vi "全局 1.vi"() -> ()   [LabVIEW 2018]
panel:
  in  "选项卡控件":enum32{"系统", "PLC", "VISON", "Mdbus", "中英文"}(tab)
  out "Exit 2":bool
  out "Exit 1":bool
  out "产品名称0":string
  out "物料编号4":string
  out "物料编号3":string
  out "产品名称2":string
  in  "系统时间":timestamp
  out "物料编号2":string
  out "机台编号":string
  out "物料编号1":string
  out "产线编号":string
  out "Login PW":dbl[](array[numeric])=[12.34, -43.21] format="%.2f"
  out "Login":i32
  out "CCIEFB Slave IP":string="192.168.3.2"
  out "ROBOT PORT":u16 format="%08x"
  out "ROBOT IP":string
  out "PLC PORT":u16 format="%08x"
  out "PLC IP":string
  out "ini文件":path
  out "产品名称1":string
  out "Exit":bool
  out "当前档位":u16
  out "PCTOUTAC远程/本地控制":bool
  out "PCTOUTAC读取目标挡位数据完成":bool
  out "配方编号":u16
  out "动作数量":string
  out "备注":string
  out "样品编号":string
  out "零件编号":string
  out "零件名称":string
  out "项目编号":string
  out "时间":sgl
  out "1# 时间数组簇":cluster{"Time":i32[]}
  out "1# 方向数组簇":T1
  out "PCTOUTAC换挡不成功":bool
  out "PCTOUTAC换挡到位":bool
  out "PCTOUTAC正在换挡":bool
  out "PCTOUTAC急停":bool
  out "PCTOUTAC学习":bool
  out "PCTOUTAC故障":bool
  out "PCTOUTAC运行/停机":bool
  out "PCTOPLC读配方结束":bool
  out "PCTOPLC下发配方参数完成":bool
  out "PCTOPLC发送启动信号":bool
  out "PCTOPLC收到NO/OFF":bool
  out "PCTOPLC读取配方完成":bool
  out "PCTOPLC下发任务完成":bool
  out "PCTOPLC保存完成":bool
  out "PCTOPLC就绪":bool
  out "PLC状态位":T2
  out "PLC档位序号":T3
  out "PLC采集值":T4
  out "检测序号":u16
  out "PLC结果":T5
  out "PLC状态":T6
  out "力":sgl[](array[numeric]) format="%.4f"
  out "检测步骤":T7
  out "PLC检测值":T8 {"3#LED电压" format="%.2f"; "3#LED电流" format="%.2f"; "3#风门开电压" format="%.2f"; "3#风门闭电压" format="%.2f"; "3#稳定压力" format="%.1f"; "3#当前压力" format="%.1f"; "3#稳定泄漏量" format="%.2f"; "3#当前泄漏量" format="%.2f"; "2#LED电压" format="%.2f"; "2#LED电流" format="%.2f"; "2#风门开电压" format="%.2f"; "2#风门闭电压" format="%.2f"; "2#稳定压力" format="%.1f"; "2#当前压力" format="%.1f"; "2#稳定泄漏量" format="%.2f"; "2#当前泄漏量" format="%.2f"; "1#LED电压" format="%.2f"; "1#LED电流" format="%.2f"; "1#风门开电压" format="%.2f"; "1#风门闭电压" format="%.2f"; "1#稳定压力" format="%.1f"; "1#当前压力" format="%.1f"; "1#稳定泄漏量" format="%.2f"; "1#当前泄漏量" format="%.2f"}
  out "高低配":i16
  out "PLC检测参数":T9 {"INV快速变化量" format="%.2f"; "INV慢速变化量" format="%.2f"; "INV变化周期" format="%.1f"; "INV初始频率" format="%.2f"; "伺服速度" format="%.1f"; "气压稳定时间" format="%.1f"; "LED电流下限" format="%.2f"; "LED电流上限" format="%.2f"; "风门开电压下限" format="%.2f"; "风门开电压上限" format="%.2f"; "风门闭电压下限" format="%.2f"; "风门闭电压上限" format="%.2f"; "压力下限" format="%.1f"; "压力上限" format="%.1f"; "泄漏量上限" format="%.2f"; "轮盘预压力" format="%.1f"}
  out "PC状态":cluster{"PLC就绪":bool, "空动作中":bool}
  out "总测试次数":i16
  out "3#视觉检测":u16[](array[numeric])
  out "2#视觉检测":u16[](array[numeric])
  out "1#视觉检测":u16[](array[numeric])
  out "PCTOUTAC参数":i16[](array[numeric])
  out "UTACTOPLC复位到原点":bool
  out "UTACTOPLC急停":bool
  out "UTACTOPLC故障复位":bool
  out "UTACTOPLC故障":bool
  out "UTACTOPLC运行/停机":bool
  out "终止序号":i16
  out "起始序号":i16
  out "UTAC设定参数":i16[](array[numeric])
  out "C-N编辑设定参数":string[](array[string])=["Delay_Time", "Acceleration_time", "Deceleration time", "X_Upper_value", "X_Lowerr_value", "Y_Upper_value", "Y_Lowerr_value", "X_displacement", "Y_displacement", "Repeat_number", "Definite_write", "Exit"]
  out "C-N编辑配方":string[](array[string])=["Recipe_number", "Detailed_location", "Explain", "Definite_write", "Exit"]
  out "C-N远程/本地":string[](array[string])=["Remote/Local", "Remote/Local Control"]
  out "C-N当前档位":string[](array[string])=["PCTOUTAC_Current_Shifter", "Current_Shifter"]
  out "C-N目标档位":string[](array[string])=["UTACTOPC_Target_Shifter", "Target_Shifter"]
  out "C-N设置":string[](array[string])=["Set", "Exit", "Edit_Recipe", "Edit_SetParameter"]
  out "C-NDI信号":string[](array[string])=["PCTOUTAC_DI_Signal", "Run/Stop", "Breakdown", "study", "Stop", "Is_Shifter", "Shifter_Succeed", "Shifter_FaildShifter"]
  out "C-NDO信号":string[](array[string])=["UTACTOPC_DO_Signal", "Run/Stop", "Breakdown", "Breakdown_Reset", "Stop", "Reset_To_origin"]
  out "C-N项目信息":string[](array[string])=["ltem_Information", "ltem_no", "Part_Name", "Part_No", "Sample_No", "Remark", "Action_Number", "Total_Test_Number", "Set"]
  # "PCTOUTAC"
  # "PCTOPLC"
  # "UTACTOPLC"
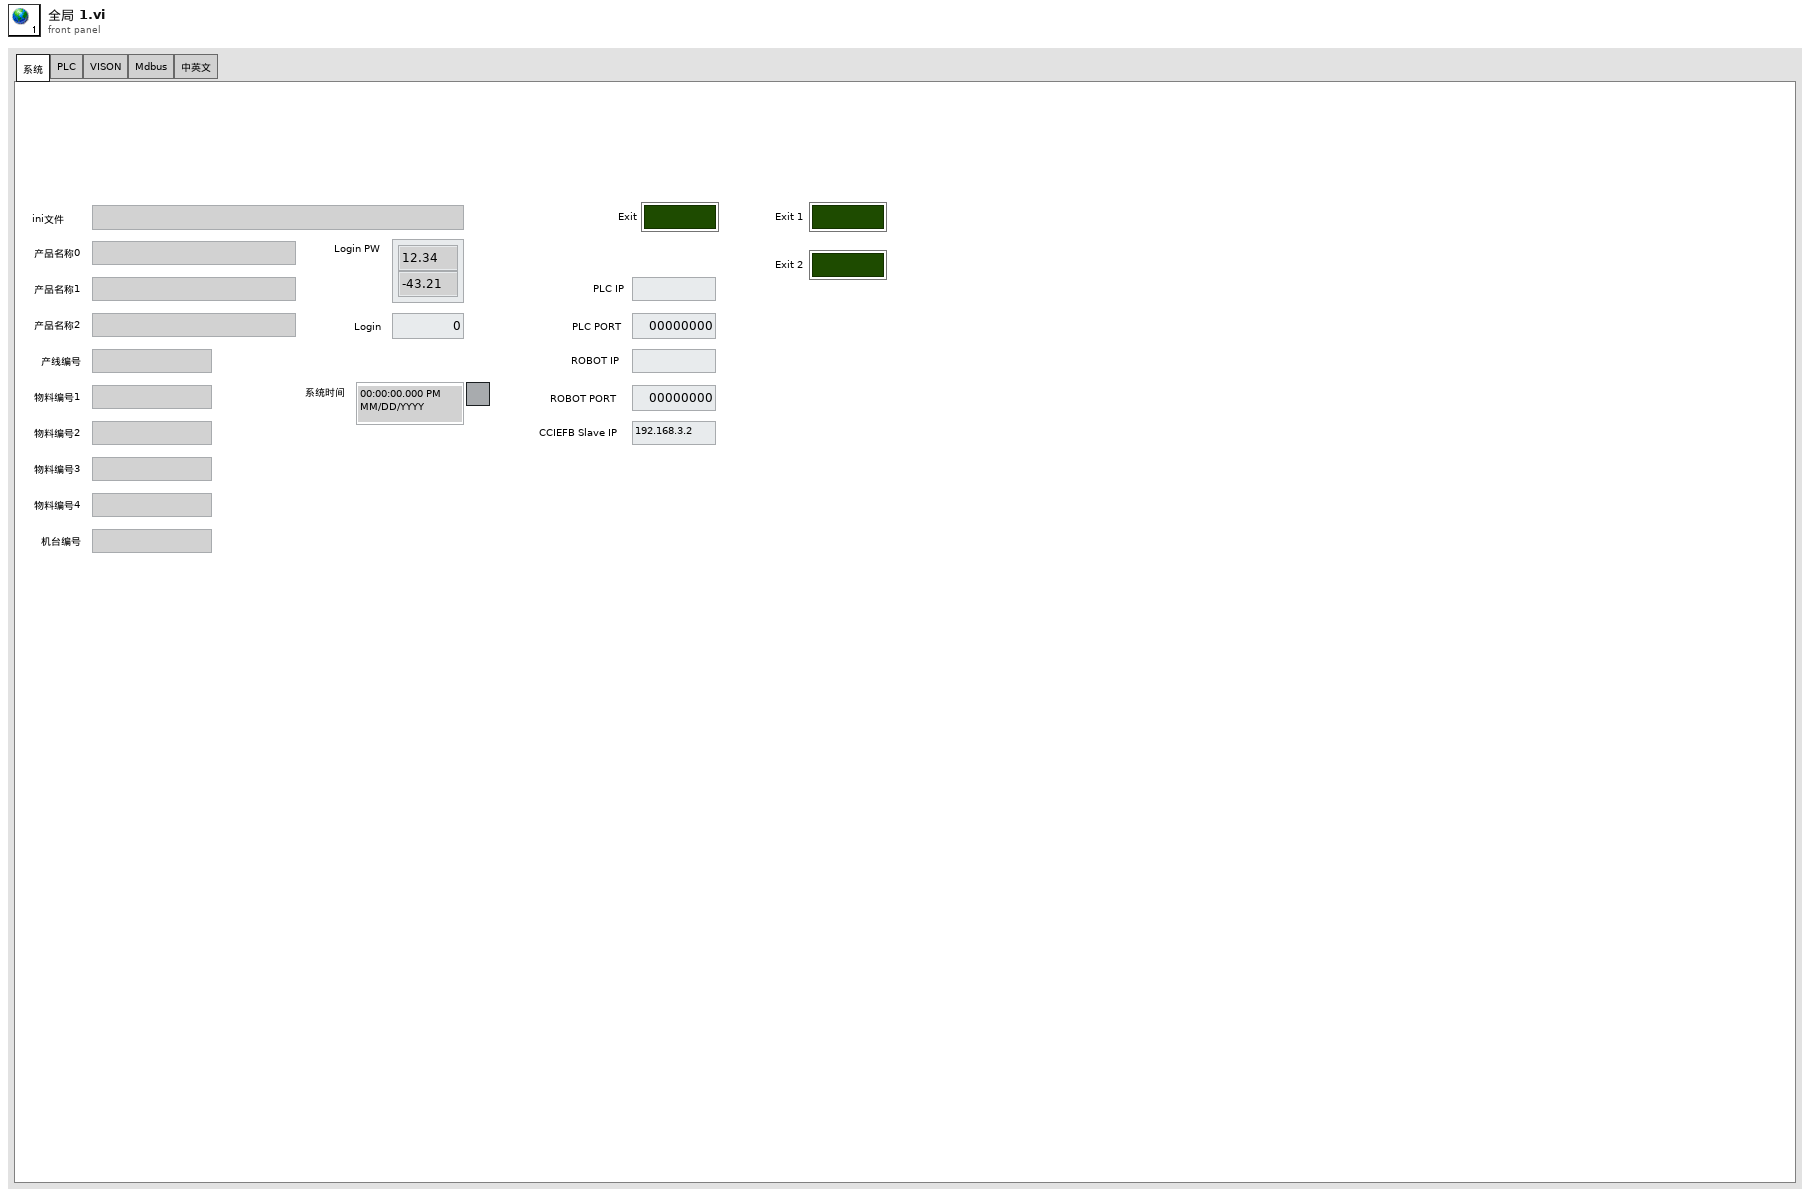
[diagram p1: front panel]
types:
  T1 = cluster{"Fx":sgl[], "Fy":sgl[], "Dx":sgl[], "Dy":sgl[]}
  T2 = cluster{"就绪":bool, "运行/停机":bool, "故障":bool, "学习":bool, "急停":bool, "正在换挡":bool, "换挡到位":bool, "换挡不成功":bool, "备用1":bool, "保存开始":bool, "等待下发任务":bool, "允许读取配方":bool, "开始采集数据":bool, "时间ON/OFF":bool, " 收到启动信号":bool, "结束采集信号":bool, "读配方参数ON/OFF":bool, "允许下发配方参数":bool}
  T3 = cluster{"挡位N1所在序号":sgl, "挡位1所在序号":sgl, "挡位N1所在序号":sgl, "挡位2所在序号":sgl, "挡位N1所在序号":sgl, " 挡位N2所在序号":sgl, "挡位3所在序号":sgl, "挡位N2所在序号":sgl, "挡位4所在序号":sgl, " 挡位N2所在序号":sgl, "挡位N3所在序号":sgl, "挡位5所在序号":sgl, "挡位N3所在序号":sgl, "挡位6所在序号":sgl, "挡位N3所在序号":sgl, "挡位N4所在序号":sgl, " 挡位7所在序号":sgl, " 挡位N4所在序号":sgl, "挡位8所在序号":sgl, "挡位N4所在序号":sgl, " 挡位N5所在序号":sgl, "挡位9所在序号":sgl, "挡位N5所在序号":sgl, " 挡位10所在序号":sgl}
  T4 = cluster{"X方向力值":sgl, "Y方向力值":sgl, "X方向位移值":sgl, "Y方向位移值":sgl}
  T5 = cluster{"1#泄漏量":bool, "1#风门闭电压":bool, "1#风门开电压":bool, "1#LED电压":bool, "1#LED电流":bool, "外观结果":bool, "2#泄漏量":bool, "2#风门闭电压":bool, "2#风门开电压":bool, "2#LED电压":bool, "2#LED电流":bool, "3#泄漏量":bool, "3#风门闭电压":bool, "3#风门开电压":bool, "3#LED电压":bool, "3#LED电流":bool}
  T6 = cluster{"PLC就绪":bool, "ROBOT就绪":bool, "空动作":bool, "检测NG":bool, "检测结束":bool, "检测开始":bool, "初始化脉冲":bool, "1#检测NG":bool, "2#检测NG":bool, "3#检测NG":bool}
  T7 = cluster{"泄漏量":bool, "风门开闭电检":bool, "LED电检":bool, "外观检测":bool, "1#轮盘关开":bool, "1#轮盘关开锁":bool, "1#轮盘开关":bool, "1#轮盘开关锁":bool, "1#拨钮左右":bool, "1#拨钮右左":bool, "1#拨钮上下":bool, "1#拨钮下上":bool, "2#轮盘关开":bool, "2#轮盘关开锁":bool, "2#轮盘开关":bool, "2#轮盘开关锁":bool, "2#拨钮左右":bool, "2#拨钮右左":bool, "2#拨钮上下":bool, "2#拨钮下上":bool, "3#轮盘关开":bool, "3#轮盘关开锁":bool, "3#轮盘开关":bool, "3#轮盘开关锁":bool, "3#拨钮左右":bool, "3#拨钮右左":bool, "3#拨钮上下":bool, "3#拨钮下上":bool}
  T8 = cluster{"1#当前泄漏量":sgl, "1#稳定泄漏量":sgl, "1#当前压力":sgl, "1#稳定压力":sgl, "1#风门闭电压":sgl, "1#风门开电压":sgl, "1#LED电流":sgl, "1#LED电压":sgl, "2#当前泄漏量":sgl, "2#稳定泄漏量":sgl, "2#当前压力":sgl, "2#稳定压力":sgl, "2#风门闭电压":sgl, "2#风门开电压":sgl, "2#LED电流":sgl, "2#LED电压":sgl, "3#当前泄漏量":sgl, "3#稳定泄漏量":sgl, "3#当前压力":sgl, "3#稳定压力":sgl, "3#风门闭电压":sgl, "3#风门开电压":sgl, "3#LED电流":sgl, "3#LED电压":sgl}
  T9 = cluster{"轮盘预压力":sgl, "泄漏量上限":sgl, "压力上限":sgl, "压力下限":sgl, "风门闭电压上限":sgl, "风门闭电压下限":sgl, "风门开电压上限":sgl, "风门开电压下限":sgl, "LED电流上限":sgl, "LED电流下限":sgl, "气压稳定时间":sgl, "伺服速度":sgl, "INV初始频率":sgl, "INV变化周期":sgl, "INV慢速变化量":sgl, "INV快速变化量":sgl}
diagram:
